vi "send calibration value loop.vi"(8 "error in (no error)":errorcluster, 10 "Address Out":string="0", 11 "VISA Refnum in":refnum<visa-resource-name>) -> (0 "error out":errorcluster, 1 "error out 2":errorcluster, 2 "Sensor On/Off Response":bool, 3 "VISA Refnum out":refnum<visa-resource-name>, 5 "Initialize/Close?":bool)   [LabVIEW 2016]
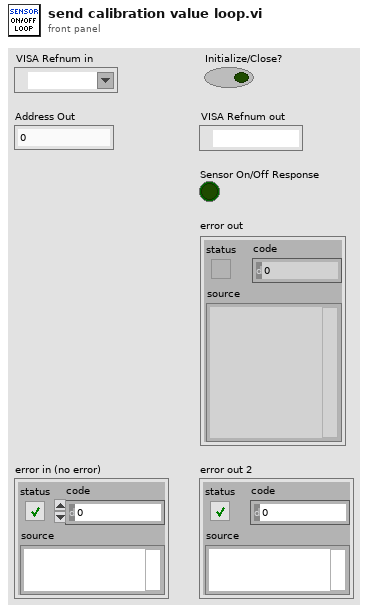
[diagram p1: front panel]
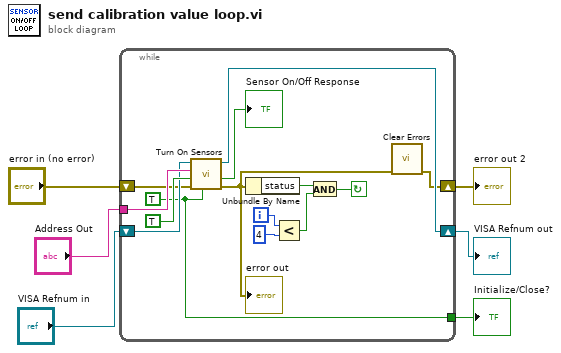
[diagram p0: block diagram]
diagram:
  n1 = while {
    tunnel: "Address Out" -> [w19]
    shift-right: [w20] -> w2
    shift-left: "VISA Refnum in" -> [w16]
    shift-right: [w7] -> w1
    shift-left: "error in (no error)" -> [w15]
    tunnel: [w9] -> w6
    i -> [w12]
    stop <- w13 continue-if-true
    w9 = TRUE ("Initialize/Close?")
    n2 = call "Turn On Sensors.vi"("Initialize/Close?"=w9, "Error In (No Error)"=w15, "Sensor On/Off"=TRUE, "Sensor Address In"=w19, "RS232 Port In"=w16) -> ("Error Out"=w8:errorcluster, "Sensor On/Off Response"=→"Sensor On/Off Response":bool, "RS232 Port Out"=w20:refnum<visa-resource-name>)  [unwired: 3 in, 1 out]
    "error out" <- w8
    n3 = Unbundle By Name(w8) -> ("status"=w14:bool)
    n4 = Less?(x=w12, y=4) -> (x < y?=w10:bool)
    n5 = And(x=w14, y=w10) -> (x .and. y?=w13:bool)
    n6 = call <vilib>:"Clear Errors.vi"("error in (no error)"=w8) -> ("error out"=w7:errorcluster)  [unwired: 5 in, 1 out]
  }
  "Initialize/Close?" <- w6
  "VISA Refnum out" <- w2
  "error out 2" <- w1
